vi "publishScanProgress.vi"(8 "error in (no error)":errorcluster, 11 "Model in":refnum<class "Model.lvclass">) -> (0 "error out":errorcluster, 3 "Model out":refnum<class "Model.lvclass">)   [LabVIEW 2015, in "Model.lvclass"]
uses:
  Model.lvclass
  Typedefs/Scan Progress.ctl
  Model.lvclass/Model.ctl
  UserEvents/UserEvents.lvclass/UserEvents.ctl
  UserEvents/UserEvents.lvclass
  Typedefs/FAMTTypedefs.lvlib
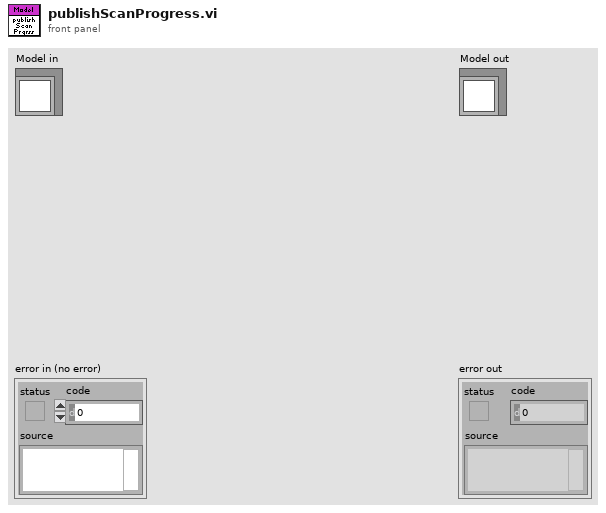
[diagram p1: front panel]
types:
  T1 = typedef "FAMTTypedefs.lvlib/Scan Progress.ctl" = cluster{"Waveform Step":u16, "Iteration":u16, "Rate Step":u16, "Amplitude Step":u16, "Waveform Total":u16, "Iteration Total":u16, "Rate Total":u16, "Amplitude Total":u16, "Current Demand":dbl[unit], "Current Rate":string, "Current Amplitude":dbl, "Actual Force":dbl[unit], "Pressure Sensor 1":dbl, "Force Error":dbl[unit]}
  T2 = typedef "ILCCommon.lvlib/ILCConfiguration.lvlib/Scan Rates.ctl" = enum16{"50", "60", "100", "120", "200", "240", "300", "400", "480", "600", "1200", "2400", "4800"}
  T3 = typedef "FAMTTypedefs.lvlib/PubDataEvents.ctl" = cluster{"State":refnum<user-event>, "ErrorCode":refnum<user-event>, "ADC Outputs":refnum<user-event>, "InputData":refnum<user-event>, "ControllerData":refnum<user-event>, "TestStatus":refnum<user-event>, "LogPath":refnum<user-event>, "ILC Outputs":refnum<user-event>, "Scan Progress":refnum<user-event>}
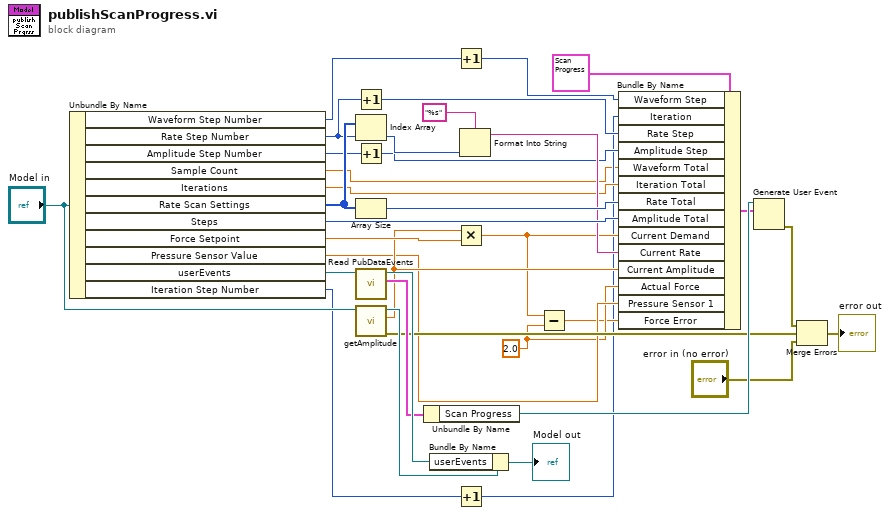
[diagram p0: block diagram]
diagram:
  w6 = dbl[unit] 2.0 ("Actual Force")
  n1 = Unbundle By Name("Model in") -> ("Waveform Step Number"=w16:u16, "Rate Step Number"=w14:u16, "Amplitude Step Number"=w12:u16, "Sample Count"=w1:dbl, "Iterations"=w4:dbl, "Rate Scan Settings"=w24:T2[], "Steps"=w23:u16, "Force Setpoint"=w10:dbl[unit], "Pressure Sensor Value"=w8:dbl, "userEvents"=w31:refnum<class "UserEvents.lvclass">, "Iteration Step Number"=w3:u16)
  n2 = Increment(x=w14) -> (x+1=w13:u16)
  n3 = Index Array(array=w24, index=w14) -> (element=w19:T2)
  n4 = Increment(x=w12) -> (x+1=w11:u16)
  n5 = Array Size(array=w24) -> (size(s)=w27:i32)
  n6 = call "Read PubDataEvents.vi"("UserEvents in"=w31) -> ("PubDataEvents"=w32:T3, "UserEvents out"=w35:refnum<class "UserEvents.lvclass">)  [unwired: 9 in]
  n7 = call "getAmplitude.vi"("Model in"="Model in") -> ("error out"=w22:errorcluster, "Result"=w9:dbl, "Model out"=w25:refnum<class "Model.lvclass">)  [unwired: 8 in]
  n8 = Unbundle By Name(w32) -> ("Scan Progress"=w33:refnum<user-event>)
  n9 = Bundle By Name(cluster=w25, "userEvents"=w35) -> (→"Model out":refnum<class "Model.lvclass">)
  n10 = Increment(x=w16) -> (x+1=w15:u16)
  n11 = Multiply(x=w9, y=w10) -> (x*y=w7:dbl[unit])
  n12 = Increment(x=w3) -> (x+1=w2:u16)
  n13 = Format Into String(format string="%s", w19) -> (resulting string=w18:string)  [unwired: 2 in, 1 out]
  n14 = Subtract(x=w7, y=w6) -> (x-y=w5:dbl[unit])
  n15 = Bundle By Name(cluster=T1 {"Waveform Step"=0, "Iteration"=0, "Rate Step"=0, "Amplitude Step"=0, "Waveform Total"=0, "Iteration Total"=0, "Rate Total"=0, "Amplitude Total"=0, "Current Demand"=0.0, "Current Rate"="", "Current Amplitude"=0.0, "Actual Force"=0.0, "Pressure Sensor 1"=0.0, "Force Error"=0.0} ("event data"), "Waveform Step"=w15, "Iteration"=w2, "Rate Step"=w13, "Amplitude Step"=w11, "Waveform Total"=w1, "Iteration Total"=w4, "Rate Total"=w27, "Amplitude Total"=w23, "Current Demand"=w7, "Current Rate"=w18, "Current Amplitude"=w9, "Actual Force"=w6, "Pressure Sensor 1"=w8, "Force Error"=w5) -> (w28:T1)
  n16 = Generate User Event(user event=w33, event data cluster=w28) -> (error out=w34:errorcluster)  [unwired: 2 in, 1 out]
  n17 = Merge Errors(w34, w22, "error in (no error)") -> (→"error out":errorcluster)
